vi "Split Description.vi"(11 "Full Description":string) -> (3 "Description":string, 5 "Hierarchy":string[](array[string]))   [LabVIEW 2020, in "VolatusGUIEditor.lvlib"]
uses:
  VolatusGUIEditor.lvlib
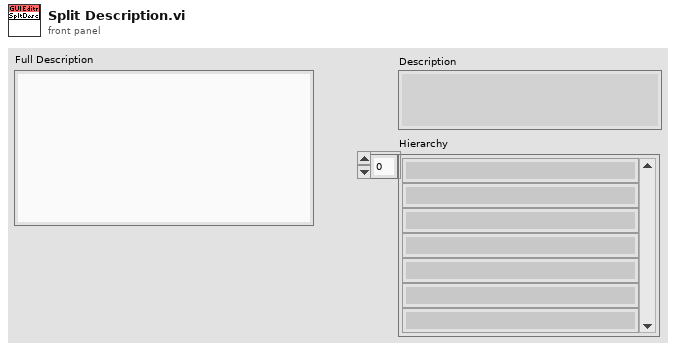
[diagram p1: front panel]
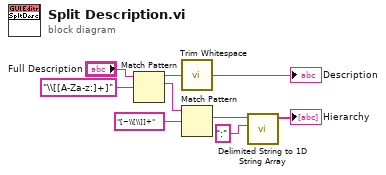
[diagram p0: block diagram]
diagram:
  n1 = Match Pattern(string="Full Description", regular expression="\\[[A-Za-z:]+]") -> (before substring=w8:string, match substring=w7:string)  [unwired: 1 in, 2 out]
  n2 = call <vilib>:"Trim Whitespace.vi"("string"=w8) -> ("trimmed string"=→"Description":string)  [unwired: 1 in]
  n3 = Match Pattern(string=w7, regular expression="[~\\[\\]]+") -> (match substring=w3:string)  [unwired: 1 in, 3 out]
  n4 = call <vilib>:"Delimited String to 1D String Array.vi"("delimiter"=":", "delimited string"=w3) -> ("string array"=→"Hierarchy":string[])  [unwired: 9 in]
